vi "RSZVB Set Tolerance.vi"(8 "error in (no error)":errorcluster {"code" format="%.0x"}, 9 "Tolerance (1.0)":dbl=1.0 format="%^.3e", 10 "Channel (1)":i32=1, 11 "VISA session":refnum<visa-resource-name>) -> (0 "error out":errorcluster {"code" format="%.0x"}, 3 "dup VISA session":refnum<visa-resource-name>)   [LabVIEW 2011]
doc: "This VI specifies the maximum deviation of the measured power from the target power of the calibration. \n\nRemote-control command(s):\nSOURce<Ch>:POWer<Pt>:CORRection:COLLect:AVERage:NTOLerance <tolerance>"
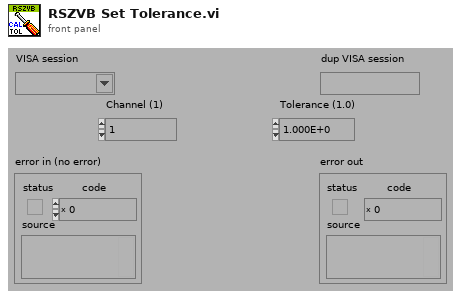
[diagram p1: front panel]
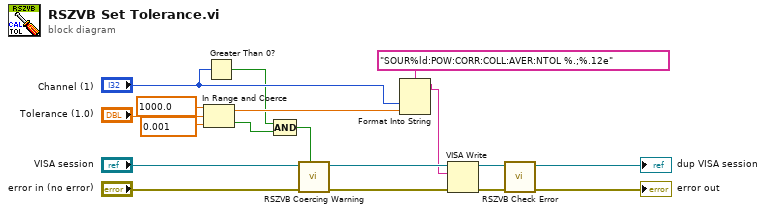
[diagram p0: block diagram]
diagram:
  n1 = In Range and Coerce(upper limit=1000.0, x="Tolerance (1.0)", lower limit=0.001) -> (coerced(x)=w4:dbl, In Range?=w2:bool)
  n2 = Greater Than 0?(x="Channel (1)") -> (x > 0?=w3:bool)
  n3 = Compound Arithmetic op=AND(w3, w2) -> (w1:bool)
  n4 = call "RSZVB Coercing Warning.vi"("In Range?"=w1, "error in (no error)"="error in (no error)", "VISA session"="VISA session") -> ("error out"=w17:errorcluster, "dup VISA session"=w18:refnum<visa-resource-name>)  [unwired: 7 in]
  n5 = Format Into String(format string="SOUR%ld:POW:CORR:COLL:AVER:NTOL %.;%.12e", "Channel (1)", w4) -> (resulting string=w13:string)  [unwired: 2 in, 1 out]
  n6 = VISA Write(VISA resource name=w18, write buffer=w13, error in (no error)=w17) -> (VISA resource name out=w15:refnum<visa-resource-name>, error out=w16:errorcluster)  [unwired: 1 out]
  n7 = call "RSZVB Check Error.vi"("error in (no error)"=w16, "VISA session"=w15) -> ("error out"=→"error out":errorcluster, "dup VISA session"=→"dup VISA session":refnum<visa-resource-name>)  [unwired: 8 in]
